vi "Initial, set and read, loop, pause (20190221) - Copy.vi"() -> ()   [LabVIEW 2017]
panel:
  in  "stop":bool
  in  "Go to wavelength":dbl
  out "Paused":bool
  in  "Pause Request":bool
  out "Message":string
  in  "Mono Wait time (ms)":u32=5000
  out "Wavelength Set":bool
  out "Total points":i32=5
  out "WL Range":dbl[](array[numeric])=[800.0, 850.0, 900.0, 950.0, 1000.0]
  in  "Step size (nm)":sgl=50.0 min=1 step=0.1
  in  "End Wavelength (nm)":dbl=1300.0 min=250.0 max=1350.0 step=0.1
  in  "Start Wavelength (nm)":dbl=500.0 min=250.0 max=1200.0 step=0.1
  out "Current wavelength":dbl=900.0
  out "Mono status":bool
  out "Output Wavelength":dbl=849.997 min=350.0 max=1100.0 step=1.0 format="%#.1f"
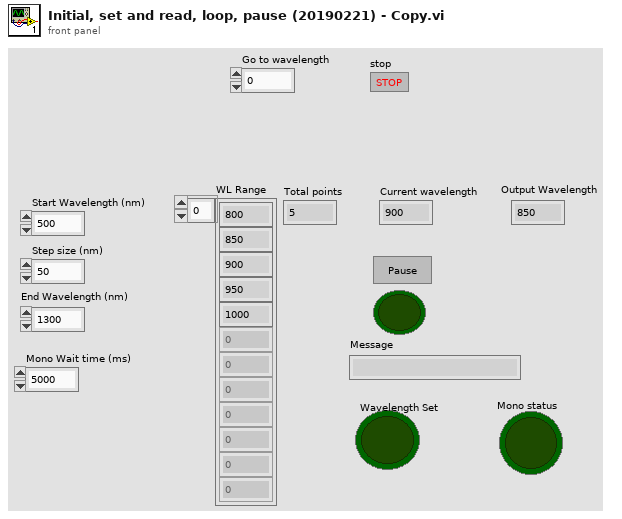
[diagram p1: front panel]
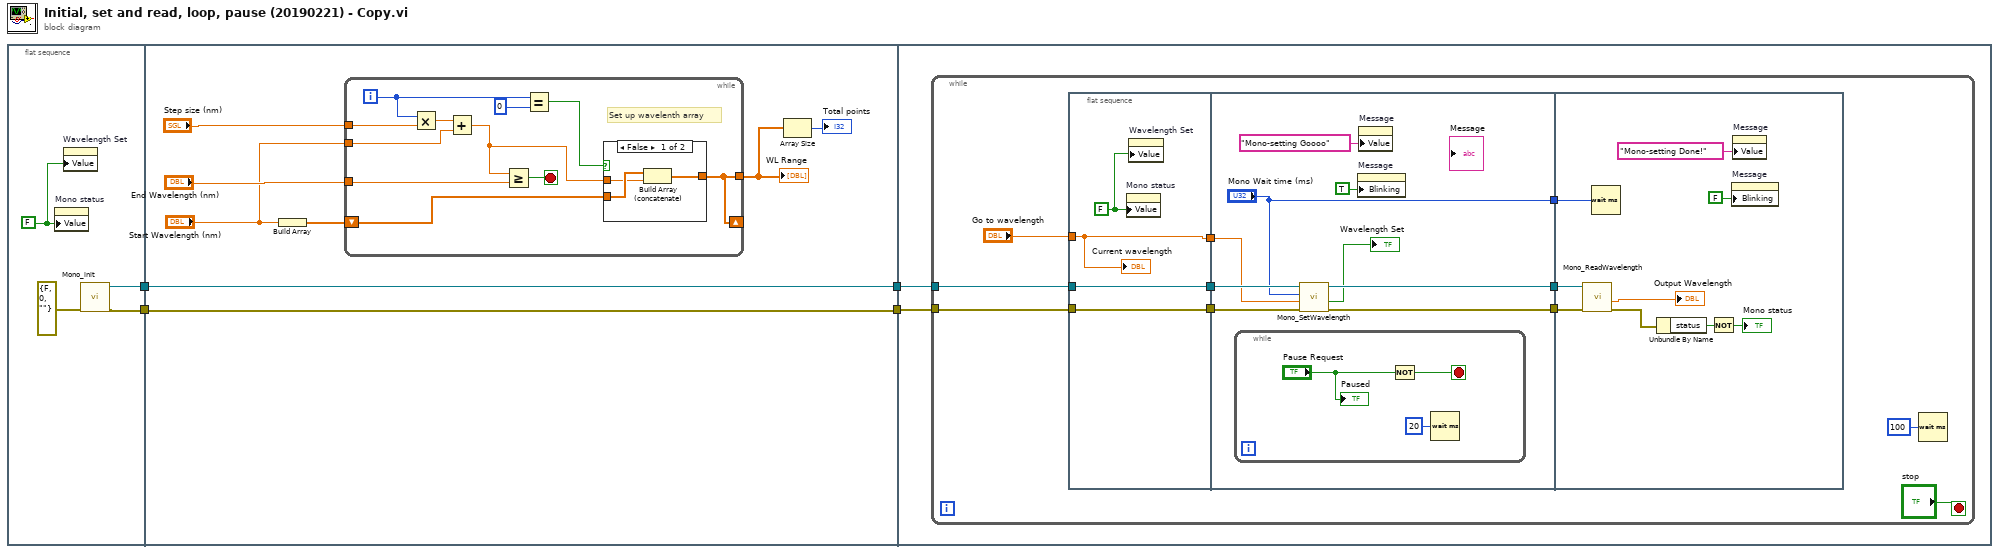
[diagram p0: block diagram]
diagram:
  n1 = flat-sequence {
    tunnel: [w7] -> w4
    tunnel: [w6] -> w2
    tunnel: w4 -> [w16]
    tunnel: [w16] -> w3
    tunnel: w2 -> [w15]
    tunnel: [w15] -> w1
    tunnel: w3 -> [w33]
    tunnel: w1 -> [w32]
    frame #0 {
      w5 = FALSE ("Mono status")
      n2 = property on="Mono status" class="Bool (strict)"("Value"=w5) -> ()  [unwired: 2 in, 2 out]
      n3 = property on="Wavelength Set" class="Bool (strict)"("Value"=w5) -> ()  [unwired: 2 in, 2 out]
      n4 = call "Mono_init.vi"("error in (no error)"=errorcluster {"status"=FALSE, "code"=0, "source"=""}) -> ("error out"=w7:errorcluster, "CmdLib"=w6:refnum<k24>)  [unwired: 8 in, 1 out]
    }
    frame #1 {
      n5 = Build Array "Build Array"("Start Wavelength (nm)") -> (w11:dbl[])
      n6 = while {
        shift-right: [w17] -> _
        shift-left: w11 -> [w19]
        tunnel: "Step size (nm)" -> [w26]
        tunnel: "End Wavelength (nm)" -> [w27]
        tunnel: "Start Wavelength (nm)" -> [w20]
        tunnel: [w17] -> w10
        i -> [w22]
        stop <- w24 stop-if-true
        # "Set up wavelenth array"
        n7 = Multiply(x=w22, y=w26) -> (x*y=w25:sgl)
        n8 = Add(x=w25, y=w20) -> (x+y=w18:dbl)
        n9 = Greater Or Equal?(x=w18, y=w27) -> (x >= y?=w24:bool)
        n10 = Equal?(x=w22, y=0) -> (x = y?=w21:bool)
        n11 = case shown="False" w21 {
          tunnel: w19 -> [w30 w31]
          tunnel: w18 -> [w29 _]
          tunnel: [w28 w31] -> w17
          frame False {
            n12 = Build Array (concatenate)(w30, w29) -> (w28:dbl[])
          }
          frame True {
          }
        }
      }
      "WL Range" <- w10
      n13 = Array Size(array=w10) -> (size(s)=→"Total points":i32)
    }
    frame #2 {
      n14 = while {
        tunnel: w33 -> [w38]
        tunnel: w32 -> [w37]
        stop <- "stop" stop-if-true
        n15 = flat-sequence {
          tunnel: "Go to wavelength" -> [w48]
          tunnel: w37 -> [w47]
          tunnel: w38 -> [w46]
          tunnel: [w48] -> w44
          tunnel: [w47] -> w43
          tunnel: [w46] -> w42
          tunnel: w44 -> [w55]
          tunnel: w43 -> [w56]
          tunnel: w42 -> [w57]
          tunnel: [w54] -> w40
          tunnel: [w53] -> w41
          tunnel: ["Mono Wait time (ms)"] -> w39
          tunnel: w41 -> [w64]
          tunnel: w40 -> [w65]
          tunnel: w39 -> [w62]
          frame #0 {
            w45 = FALSE ("Mono status")
            n16 = property on="Mono status" class="Bool (strict)"("Value"=w45) -> ()  [unwired: 2 in, 2 out]
            n17 = property on="Wavelength Set" class="Bool (strict)"("Value"=w45) -> ()  [unwired: 2 in, 2 out]
            "Current wavelength" <- w48
          }
          frame #1 {
            n18 = while {
              stop <- w59 stop-if-true
              n19 = Not(x="Pause Request") -> (.not. x?=w59:bool)
              n20 = Wait (ms)(milliseconds to wait=u32 20) -> ()  [unwired: 1 out]
              "Paused" <- "Pause Request"
            }
            n21 = call "Mono_SetWavelength.vi"("error in (no error) 2"=w57, "Wavelength"=w55, "Mono Wait time (ms)"="Mono Wait time (ms)", "CmdLib In"=w56) -> ("error out 2"=w54:errorcluster, "Wavelength Set"=→"Wavelength Set":bool, "CmdLib Out"=w53:refnum<k24>)  [unwired: 5 in]
            n22 = property on="Message" class="Str"("Blinking"=TRUE) -> ()  [unwired: 2 in, 2 out]
            n23 = property on="Message" class="Str"("Value"="Mono-setting Goooo" ("Message")) -> ()  [unwired: 2 in, 2 out]
          }
          frame #2 {
            n24 = call "Mono_ReadWavelength.vi"("error in (no error) 2"=w65, "CmdLib In"=w64) -> ("error out 2"=w66:errorcluster, "getWavelength"=→"Output Wavelength":dbl)  [unwired: 7 in, 1 out]
            n25 = Wait (ms)(milliseconds to wait=w62) -> ()  [unwired: 1 out]
            n26 = Unbundle By Name(w66) -> ("status"=w68:bool)
            n27 = Not(x=w68) -> (.not. x?=→"Mono status":bool)
            n28 = property on="Message" class="Str"("Blinking"=FALSE) -> ()  [unwired: 2 in, 2 out]
            n29 = property on="Message" class="Str"("Value"="Mono-setting Done!" ("Message")) -> ()  [unwired: 2 in, 2 out]
          }
        }
        n30 = Wait (ms)(milliseconds to wait=u32 100) -> ()  [unwired: 1 out]
      }
    }
  }
